vi "Enqueue Request Message.vi"(8 "error in (no error)":errorcluster, 9 "Message Data":variant, 10 "Message":string, 11 "Process In":refnum<class "Process.lvclass">) -> (0 "error out":errorcluster, 3 "Process Out":refnum<class "Process.lvclass">)   [LabVIEW 2020, in "Process.lvclass"]
doc: "For a regular message, enqueue the message. For a priority message, enqueue it at the front of the queue."
uses:
  Process.lvclass
  Process.lvclass/Process.ctl
  Protected/Messaging/Request Message Cluster.ctl
  Protected/Messaging/Message Cluster.ctl
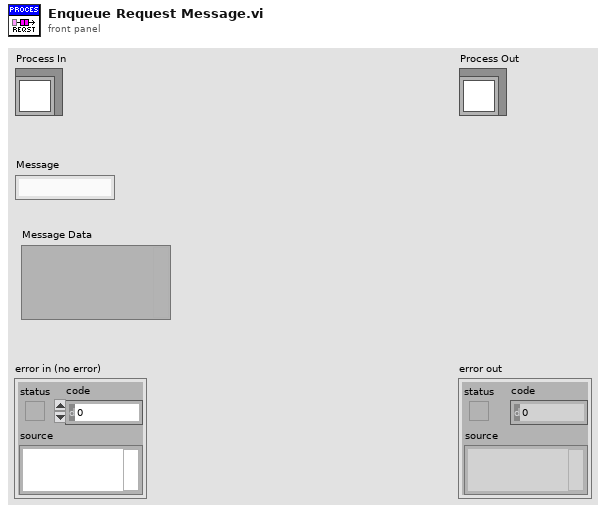
[diagram p1: front panel]
types:
  T1 = typedef "Process.lvclass/Request Message Cluster.ctl" = cluster{"Message":string, "Message Data":variant, "Request Error":errorcluster}
  T2 = typedef "Process.lvclass/Message Cluster.ctl" = cluster{"Message":string, "Message Data":variant, "Request Notifier":refnum<notifier>}
  T3 = cluster{"Action":string, "Call Chain":string, "Process":string, "Message":string, "Message Data":variant, "Time":u32}
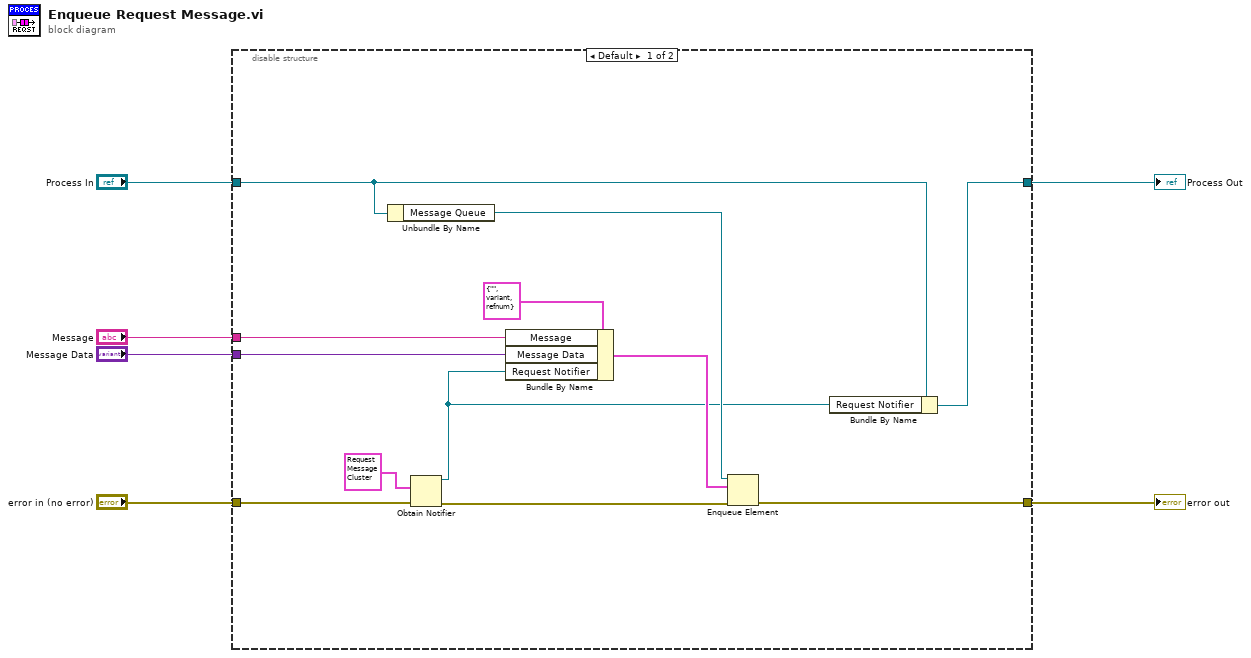
[diagram p0: block diagram]
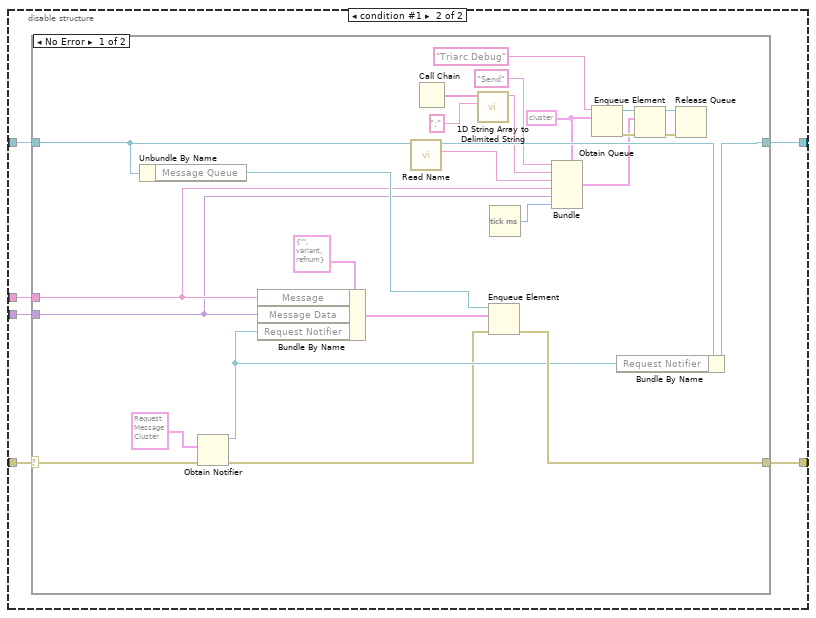
[diagram p2: hidden frame]
diagram:
  n1 = disable-structure shown="Default" {
    disable-tunnel: "Process In" -> [w7 w22]
    disable-tunnel: "error in (no error)" -> [w10 w24]
    disable-tunnel: [w17 w23] -> w4
    disable-tunnel: "Message Data" -> [w16 w19]
    disable-tunnel: "Message" -> [w15 w20]
    disable-tunnel: [w8 w21] -> w1
    frame condition #0 (active) {
      n2 = Unbundle By Name(w7) -> ("Message Queue"=w18:refnum<queue>)
      n3 = Obtain Notifier(notification data type=T1 {"Message"="", "Message Data"=variant, "Request Error"={"status"=FALSE, "code"=0, "source"=""}} ("Message Cluster"), error in (no error)=w10) -> (notifier out=w11:refnum<notifier>, error out=w9:errorcluster)  [unwired: 2 in, 1 out]
      n4 = Bundle By Name(cluster=T2 {"Message"="", "Message Data"=variant, "Request Notifier"=refnum} ("Message Cluster"), "Message"=w15, "Message Data"=w16, "Request Notifier"=w11) -> (w14:T2)
      n5 = Enqueue Element(queue=w18, element=w14, error in (no error)=w9) -> (error out=w17:errorcluster)  [unwired: 1 in, 2 out]
      n6 = Bundle By Name(cluster=w7, "Request Notifier"=w11) -> (w8:refnum<class "Process.lvclass">)
    }
    frame condition #1 {
      n7 = case shown="No Error" w24 {
        selector: w24 -> [w26 w51]
        tunnel: [w47 w51] -> w23
        tunnel: w22 -> [w46 w52]
        tunnel: [w29 w52] -> w21
        tunnel: w20 -> [w43 _]
        tunnel: w19 -> [w42 _]
        frame No Error {
          w37 = T3 {"Action"="", "Call Chain"="", "Process"="", "Message"="", "Message Data"=variant, "Time"=0} ("output cluster")
          n8 = Unbundle By Name(w46) -> ("Message Queue"=w50:refnum<queue>)
          n9 = Obtain Notifier(notification data type=T1 {"Message"="", "Message Data"=variant, "Request Error"={"status"=FALSE, "code"=0, "source"=""}} ("Message Cluster"), error in (no error)=w26) -> (notifier out=w27:refnum<notifier>, error out=w25:errorcluster)  [unwired: 2 in, 1 out]
          n10 = Bundle By Name(cluster=T2 {"Message"="", "Message Data"=variant, "Request Notifier"=refnum} ("Message Cluster"), "Message"=w43, "Message Data"=w42, "Request Notifier"=w27) -> (w49:T2)
          n11 = call "Read Name.vi"("Process In"=w46) -> ("Qualified Name"=w44:string, "Process Out"=w45:refnum<class "Process.lvclass">)  [unwired: 7 in, 2 out]
          n12 = Call Chain() -> (call chain=w41:string[])
          n13 = call <vilib>:"1D String Array to Delimited String.vi"("delimiter"=":", "string array"=w41) -> ("delimited string"=w39:string)  [unwired: 9 in]
          n14 = Enqueue Element(queue=w50, element=w49, error in (no error)=w25) -> (error out=w47:errorcluster)  [unwired: 1 in, 2 out]
          n15 = Tick Count (ms)() -> (millisecond timer value=w30:u32)
          n16 = Bundle(cluster=w37, "Action"="Send", "Call Chain"=w39, "Process"=w44, "Message"=w43, "Message Data"=w42, "Time"=w30) -> (w34:T3)
          n17 = Obtain Queue(name (unnamed)="Triarc Debug", element data type=w37) -> (queue out=w36:refnum<queue>, error out=w35:errorcluster)  [unwired: 3 in, 1 out]
          n18 = Bundle By Name(cluster=w45, "Request Notifier"=w27) -> (w29:refnum<class "Process.lvclass">)
          n19 = Enqueue Element(queue=w36, element=w34, error in (no error)=w35) -> (queue out=w33:refnum<queue>, error out=w32:errorcluster)  [unwired: 1 in, 1 out]
          n20 = Release Queue(queue=w33, error in (no error)=w32) -> ()  [unwired: 1 in, 3 out]
        }
        frame Error {
        }
      }
    }
  }
  "error out" <- w4
  "Process Out" <- w1
